vi "emg_robot_control.vi"() -> ()   [LabVIEW 2023]
uses:
  <vilib>/MakerHub/LINX/Public/Peripherals/Analog/Analog Read 1 Chan.vi
  <vilib>/MakerHub/LINX/Public/Peripherals/Analog/Analog Read N Chans.vi
  <vilib>/MakerHub/LINX/Private/Local IO/LinxAnalogRead.vi
  <vilib>/MakerHub/LINX/Public/Utilities/Check Channel.vi
  <vilib>/MakerHub/LINX/Public/Utilities/Open Serial.vi
  <vilib>/MakerHub/LINX/Public/Sensors/Motion/Servo/Servo Open N Channels.vi
  <vilib>/MakerHub/LINX/Public/Sensors/Motion/Servo/Servo Set Pulse Width One Channel.vi
  <vilib>/MakerHub/LINX/Private/Utilties/Generate Error.vi
  <vilib>/MakerHub/LINX/Public/Sensors/Motion/Servo/Servo Close N Channels.vi
  <vilib>/MakerHub/LINX/LMH-LINX.lvlib
  <vilib>/MakerHub/LINX/Public/Sensors/Motion/Servo/Servo.lvlib
panel:
  out "Speed or no speed":i32
  out "Position of each servo":u8[](array[numeric])
  out "index of element":i32
  out "appended array":u16[](array[numeric])
  in  "array":u8[](array[numeric])
  out "Current Position":i32
  out "Error Out 2":errorcluster
  out "Servo chosen":u8
  out "Previous State":dbl
  out "Processed Signal":dbl(graph)
  in  "Stop programme":bool
  out "Error Out":errorcluster
  in  "Serial Port":refnum<visa-resource-name>="N/A"
  out "Loop Rate (Hz)":u32
  out "Raw Signal":dbl(graph)
  in  "Analog Input Channel":u8=13
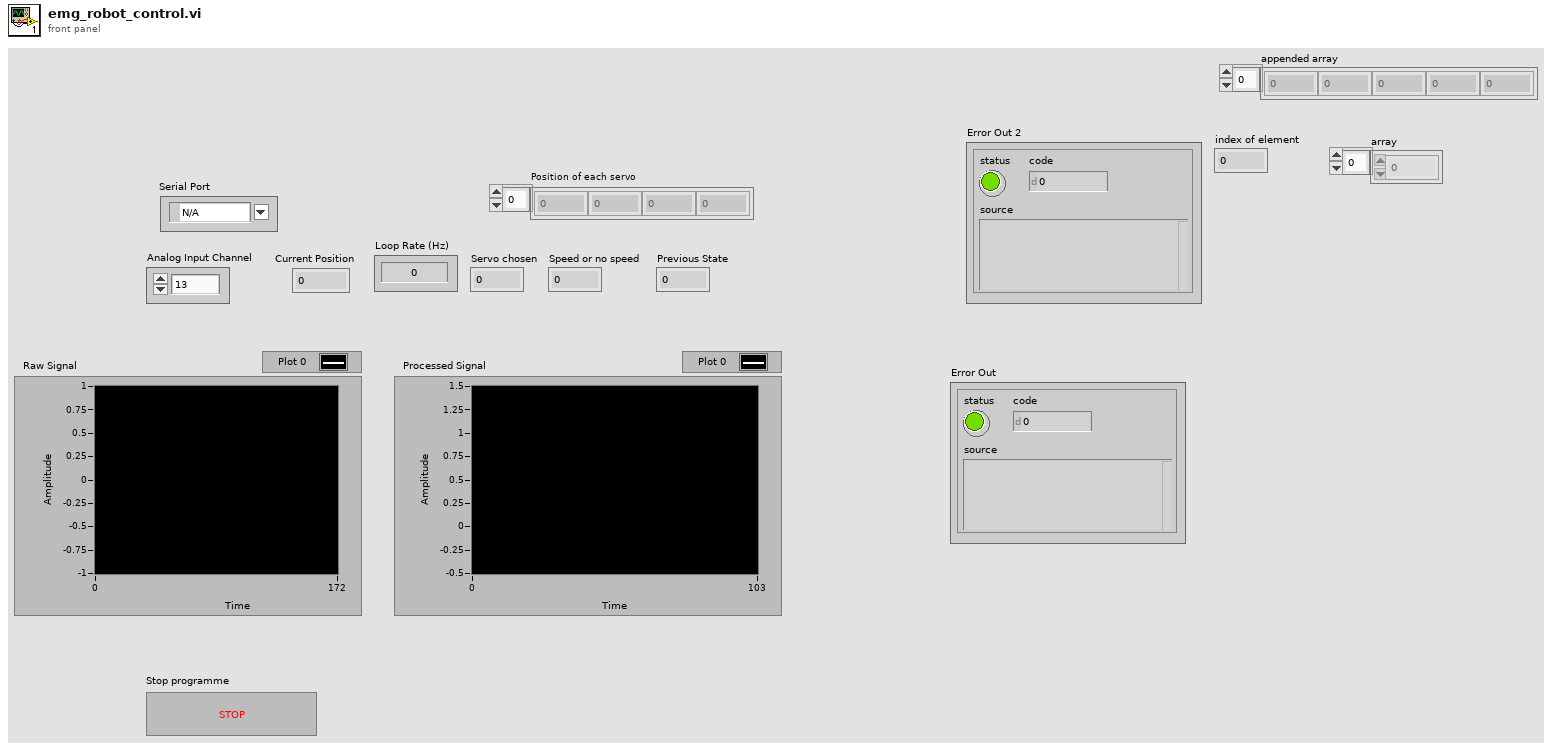
[diagram p1: front panel]
types:
  T1 = typedef "LMH-LINX.lvlib/LINX Ref.ctl" = cluster{"IO":T2, "Interface":T3, "LINX Device Config":T4}
  T2 = typedef "LMH-LINX.lvlib/Platform.ctl" = enum16{"Remote", "Local"}
  T3 = typedef "LMH-LINX.lvlib/Interface.ctl" = enum16{"Serial", "TCP"}
  T4 = typedef "LMH-LINX.lvlib/Device.lvlib/LINX Device Config.ctl" = cluster{"Interface":T3, "COM Port":refnum<visa-resource-name>, "TCP Configuration":T5, "Device Family":u8, "Device ID":u8, "Device Name":string, "TCP Ref":refnum<k5>, "Channels":T6}
  T5 = typedef "LMH-LINX.lvlib/Device.lvlib/TCP Config.ctl" = cluster{"IP Address":string, "Port":u16}
  T6 = typedef "LMH-LINX.lvlib/Channels.ctl" = cluster{"DI":u8[], "DO":u8[], "AI":u8[], "AO":u8[], "PWM":u8[], "QE":u8[], "UART":u8[], "I2C 2":u8[], "SPI":u8[], "CAN":u8[], "Servo":u8[], "AI Ref (V)":dbl, "AI Resolution (Bits)":u8, "AO Ref (V)":dbl, "AO Resolution (Bits)":u8}
  T7 = cluster{"[0]":i32, "[1]":i32, "[2]":i32, "[3]":i32, "[4]":i32, "[5]":i32, "[6]":i32, "[7]":i32, "[8]":i32}
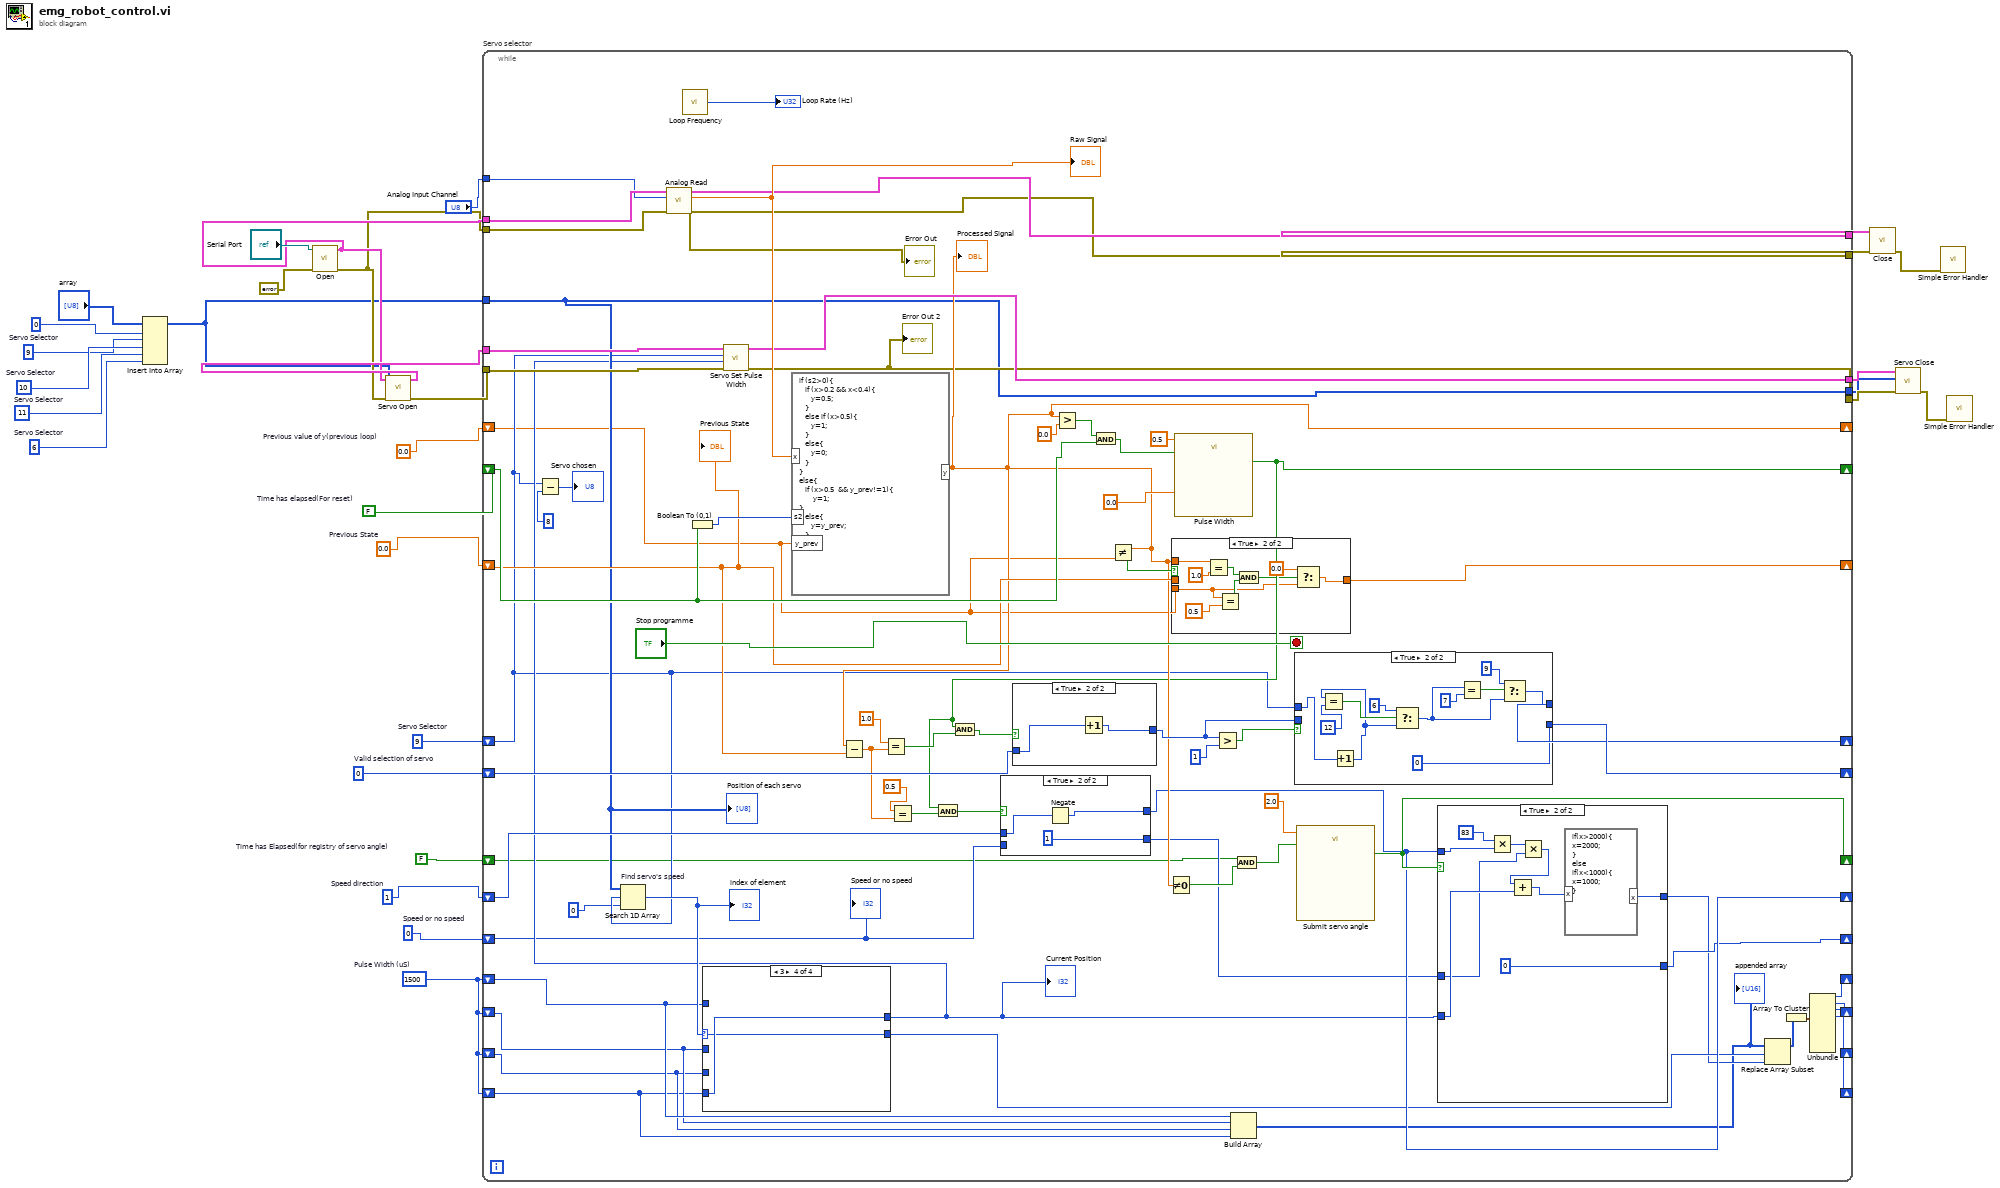
[diagram p0: block diagram]
diagram:
  w5 = u8 6  # Servo Selector
  w6 = u8 11  # Servo Selector
  w7 = u8 9  # Servo Selector
  w8 = u8 10  # Servo Selector
  w1 = u16 0  # Speed or no speed
  w10 = i16 1  # Speed direction
  w9 = 1500  # Pulse Width (uS)
  w11 = FALSE  # Time has Elapsed(for registry of servo angle)
  w12 = 0  # Valid selection of servo
  w13 = FALSE  # Time has elapsed(For reset)
  w16 = 0.0  # Previous State
  w17 = 0.0  # Previous value of y(previous loop)
  w19 = u8 9  # Servo Selector
  n1 = Insert Into Array(array="array", index=0, new element #1=w7, new element #2=w8, new element #3=w6, new element #4=w5) -> (w2:u8[])
  n2 = call-poly <vilib>:"Open.vi"("Error In"=errorcluster {"status"=FALSE, "code"=0, "source"=""}, "Serial Port"="Serial Port") -> ("Error Out"=w14:errorcluster, "LINX Resource"=w15:T1)  [unwired: 7 in, 1 out]
  n3 = call-poly <vilib>:"Servo Open.vi"("Error In"=w14, "Servo Channels"=w2, "LINX Resource"=w15) -> ("Error Out"=w23:errorcluster, "LINX Resource"=w25:T1)  [unwired: 7 in]
  n4 = while "Servo selector" {
    tunnel: w15 -> [w98]
    tunnel: [w76] -> w29
    tunnel: w14 -> [w97]
    tunnel: [w75] -> w30
    tunnel: "Analog Input Channel" -> [w95]
    tunnel: w25 -> [w93]
    tunnel: [w92] -> w24
    tunnel: w23 -> [w91]
    tunnel: [w55] -> w22
    shift-right: [w70] -> _
    shift-left: w19 -> [w36]
    shift-right: [w64] -> _
    shift-left: w17 -> [w31]
    shift-right: [w81] -> _
    shift-left: w16 -> [w80]
    tunnel: [w53] -> w18
    tunnel: w2 -> [w53]
    shift-right: [w59] -> _
    shift-left: w13 -> [w84]
    shift-right: [w71] -> _
    shift-left: w12 -> [w73]
    shift-right: [w63] -> _
    shift-left: w11 -> [w32]
    shift-right: [w44] -> _
    shift-left: w9 -> [w51]
    shift-right: [w56] -> _
    shift-left: w10 -> [w57]
    shift-right: [w43] -> _
    shift-left: w9 -> [w50]
    shift-right: [w42] -> _
    shift-left: w9 -> [w49]
    shift-right: [w33] -> _
    shift-left: w9 -> [w48]
    shift-right: [w39] -> _
    shift-left: w1 -> [w40]
    stop <- "Stop programme" stop-if-true
    n5 = Subtract(x=w36, y=u8 8) -> (x-y=→"Servo chosen":u8)
    n6 = Search 1D Array "Find servo's speed"(1D array=w53, element=w36, start index (0)=u8 0) -> (index of element=w52:i32)
    "index of element" <- w52
    n7 = call-poly <vilib>:"Analog Read.vi"("Error In"=w97, "Analog Channel"=w95, "LINX Resource"=w98) -> ("Error Out"=w75:errorcluster, "Voltage"=w94:dbl, "LINX Resource"=w76:T1)  [unwired: 5 in, 1 out]
    "Raw Signal" <- w94
    "Error Out" <- w75
    n8 = call <vilib>:"Loop Frequency.vi"() -> ("Loop Rate (Hz)"=→"Loop Rate (Hz)":u32)
    n9 = Boolean To (0,1)(Boolean=w84) -> (0, 1=w83:i16)
    n10 = case shown="3" w52 {
      selector: w52 -> [w99 w101 w103 w105]
      tunnel: w51 -> [w100 _ _ _]
      tunnel: [w100 w102 w104 w106] -> w41
      tunnel: w50 -> [_ w102 _ _]
      tunnel: w49 -> [_ _ w104 _]
      tunnel: w48 -> [_ _ _ w106]
      tunnel: [w99 w101 w103 w105] -> w47
      frame 0, Default {
      }
      frame 1 {
      }
      frame 2 {
      }
      frame 3 {
      }
    }
    "Current Position" <- w41
    n11 = call-poly <vilib>:"Servo Set Pulse Width.vi"("Error In"=w91, "Pulse Width (uS)"=w41, "Servo Channel"=w36, "LINX Resource"=w93) -> ("Error Out"=w55:errorcluster, "LINX Resource"=w92:T1)  [unwired: 6 in]
    "Error Out 2" <- w55
    n12 = formula code="if (s2>0){\n   if (x>0.2 && x<0.4){\n      y=0.5;\n   }\n   else if (x>0.5){\n      y=1;\n   }\n   else{\n      y=0;\n   }\n}\nelse{\n   if (x>0.5  && y_prev!=1){\n       y=1;\n}\n   else{\n      y=y_prev;\n   }\n}"("x"=w94, "y_prev"=w31, "s2"=w83) -> ("y"=w64:dbl)
    "Processed Signal" <- w64
    n13 = Subtract(x=w64, y=w80) -> (x-y=w62:dbl)
    n14 = Equal?(x=1.0, y=w62) -> (x = y?=w79:bool)
    n15 = Equal?(x=0.5, y=w62) -> (x = y?=w60:bool)
    n16 = Greater?(x=w64, y=0.0) -> (0:w86:bool)
    n17 = And(x=w86, y=w84) -> (x .and. y?=w85:bool)
    n18 = Not Equal?(x=w64, y=w31) -> (x != y?=w82:bool)
    n19 = Not Equal To 0?(x=w64) -> (x != 0?=w65:bool)
    n20 = case shown="True" w82 {
      tunnel: [w139 w140] -> w81
      tunnel: w80 -> [w139 _]
      tunnel: w31 -> [_ w141]
      tunnel: w64 -> [_ w146]
      frame False {
      }
      frame True {
        n21 = Equal?(x=w146, y=1.0) -> (x = y?=w144:bool)
        n22 = Equal?(x=w141, y=0.5) -> (x = y?=w147:bool)
        n23 = And(x=w144, y=w147) -> (x .and. y?=w143:bool)
        n24 = Select(t=0.0, s=w143, f=w141) -> (s? t:f=w140:dbl)
      }
    }
    n25 = call "Pulse Width"("Time Target (s)"=0.5, "Reset"=w85, "Set Start Time (s)"=0.0) -> ("Time has Elapsed"=w59:bool)  [unwired: 9 in, 7 out]
    n26 = And(x=w59, y=w60) -> (x .and. y?=w58:bool)
    n27 = And(x=w59, y=w79) -> (x .and. y?=w54:bool)
    n28 = case shown="True" w58 {
      tunnel: w57 -> [w108 w111]
      tunnel: [w108 w110] -> w56
      tunnel: w40 -> [w107 _]
      tunnel: [w107 i16 1] -> w38
      frame False {
      }
      frame True {
        n29 = Negate(x=w111) -> (-x=w110:i16)
      }
    }
    n30 = case shown="True" w54 {
      tunnel: w73 -> [w136 w138]
      tunnel: [w136 w137] -> w67
      frame False {
      }
      frame True {
        n31 = Increment(x=w138) -> (x+1=w137:i32)
      }
    }
    n32 = Greater?(x=w67, y=1) -> (0:w72:bool)
    n33 = Build Array(w51, w50, w49, w48) -> (w34:i32[])
    "appended array" <- w34
    n34 = And(x=w32, y=w65) -> (x .and. y?=w66:bool)
    n35 = case shown="True" w72 {
      tunnel: [w124 0] -> w71
      tunnel: w67 -> [w124 _]
      tunnel: w36 -> [w123 w131]
      tunnel: [w123 w126] -> w70
      frame False {
      }
      frame True {
        n36 = Increment(x=w131) -> (x+1=w130:u8)
        n37 = Equal?(x=w130, y=u8 12) -> (x = y?=w134:bool)
        n38 = Select(t=u8 6 ("y"), s=w134, f=w130) -> (s? t:f=w127:u8)
        n39 = Equal?(x=w127, y=u8 7) -> (x = y?=w128:bool)
        n40 = Select(t=u8 9 ("y"), s=w128, f=w127) -> (s? t:f=w126:u8)
      }
    }
    n41 = call "Submit servo angle"("Time Target (s)"=2.0, "Reset"=w66) -> ("Time has Elapsed"=w63:bool)  [unwired: 10 in, 7 out]
    n42 = case shown="True" w63 {
      tunnel: w41 -> [w112 w120]
      tunnel: w56 -> [_ w122]
      tunnel: w38 -> [w113 w116]
      tunnel: [w113 0] -> w39
      tunnel: [w112 w115] -> w37
      frame False {
      }
      frame True {
        n43 = Multiply(x=i16 83, y=w122) -> (x*y=w117:i16)
        n44 = Multiply(x=w117, y=w116) -> (x*y=w114:i32)
        n45 = Add(x=w114, y=w120) -> (x+y=w119:i16)
        n46 = formula code="if(x>2000){\nx=2000;\n}\nelse if(x<1000){\nx=1000;\n}"("x"=w119) -> ("x"=w115:i16)
      }
    }
    n47 = Replace Array Subset(array=w34, new element=w37, index=w47) -> (w46:i32[])
    n48 = Array To Cluster(array=w46) -> (cluster=w45:T7)
    n49 = Unbundle(w45) -> ("[0]"=w44:i32, "[1]"=w43:i32, "[2]"=w42:i32, "[3]"=w33:i32)  [unwired: 5 out]
    "Previous State" <- w80
    "Position of each servo" <- w53
    "Speed or no speed" <- w40
  }
  n50 = call <vilib>:"Close.vi"("Error In"=w30, "LINX Resource"=w29) -> ("Error Out"=w21:errorcluster)  [unwired: 9 in]
  n51 = call-poly <vilib>:"Servo Close.vi"("Error In"=w22, "Servo Channels"=w18, "LINX Resource"=w24) -> ("Error Out"=w20:errorcluster)  [unwired: 7 in, 1 out]
  n52 = call <vilib>:"Simple Error Handler.vi"("error in (no error)"=w21) -> ()  [unwired: 4 in, 5 out]
  n53 = call <vilib>:"Simple Error Handler.vi"("error in (no error)"=w20) -> ()  [unwired: 4 in, 5 out]
